vi "slider from labview.vi"() -> ()   [LabVIEW 2020]
uses:
  <vilib>/Instr/_visa.llb/VISA Configure Serial Port (Instr).vi
panel:
  in  "stop":bool
  in  "VISA resource name":refnum<visa-resource-name>
  in  "Slide":dbl(slide) scale=-40.0..40.0
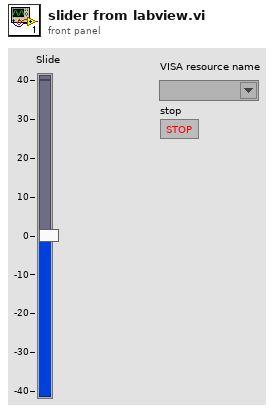
[diagram p1: front panel]
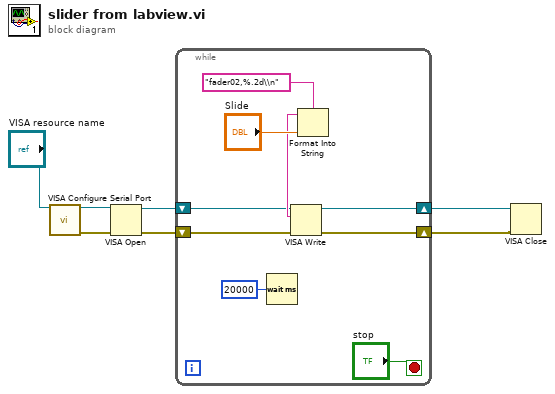
[diagram p0: block diagram]
diagram:
  n1 = call-poly "VISA Configure Serial Port"("VISA resource name"="VISA resource name") -> ("VISA resource name out"=w3:refnum<visa-resource-name>, "error out"=w2:errorcluster)  [unwired: 13 in]
  n2 = VISA Open(error in (no error)=w2, VISA resource name=w3) -> (VISA resource name=w7:refnum<visa-resource-name>, error out=w6:errorcluster)  [unwired: 3 in]
  n3 = while {
    shift-right: [w11] -> w5
    shift-left: w7 -> [w13]
    shift-right: [w10] -> w4
    shift-left: w6 -> [w12]
    stop <- "stop" stop-if-true
    n4 = Wait (ms)(milliseconds to wait=u32 20000) -> ()  [unwired: 1 out]
    n5 = Format Into String(format string="fader02,%.2d\\n", "Slide") -> (resulting string=w14:string)  [unwired: 2 in, 1 out]
    n6 = VISA Write(VISA resource name=w13, write buffer=w14, error in (no error)=w12) -> (VISA resource name out=w11:refnum<visa-resource-name>, error out=w10:errorcluster)  [unwired: 1 out]
  }
  n7 = VISA Close(VISA resource name=w5, error in (no error)=w4) -> ()  [unwired: 1 out]
